vi "NGTS_DAQmx_AI Clock and Trigger.vi"(8 "error in":errorcluster, 10 "AI Tasks In":refnum<k21>) -> (0 "error out":errorcluster, 2 "AI Tasks Out":refnum<k21>)   [LabVIEW 2018]
doc: "Sets sample clock rate and starts tasks for AI\n\n2007_05 Mike Ashe\nmichael.ashe@imaginatics.net\nCell: 860-961-0876"
uses:
  <vilib>/DAQmx/configure/timing.llb/DAQmx Timing (Sample Clock).vi
panel:
  # "PXI Device Names only\nused for Complex Trigger Mode"
  # "If a value is wired here, use it.\nIf not, then use value in INI"
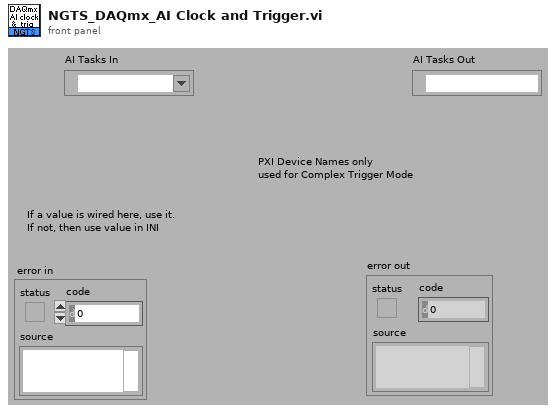
[diagram p1: front panel]
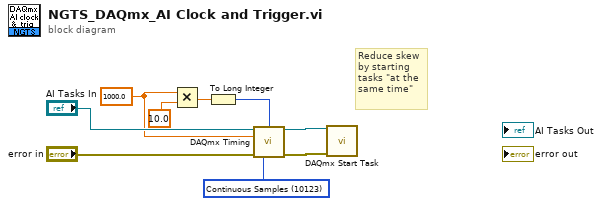
[diagram p0: block diagram]
diagram:
  w1 = 1000.0 ("rate")
  w2 = 10123 items=["Finite Samples"=10178, "Continuous Samples"=10123] ("sample mode")
  # "Reduce skew\nby starting\ntasks \"at the\nsame time\""
  n1 = Multiply(x=w1, y=10.0) -> (x*y=w4:dbl)
  n2 = To Long Integer(number=w4) -> (32bit integer=w3:i32)
  n3 = call-poly <vilib>:"DAQmx Timing.vi"("task/channels in"="AI Tasks In", "sample mode"=w2, "samples per channel"=w3, "rate"=w1, "error in"="error in") -> ("task out"=w6:refnum<k21>, "error out"=w7:errorcluster)  [unwired: 9 in]
  n4 = call <vilib>:"DAQmx Start Task.vi"("task/channels in"=w6, "error in"=w7) -> ()  [unwired: 12 in, 2 out]
